vi "ResetFlowAvgFGV.vi"(9 "ignore previous (T)":bool, 10 "timeout in ms (-1)":i32=-1, 11 "Action":enum16{"Create", "Set", "Wait"}(ring)=enum."Set") -> (2 "timed out?":bool=TRUE)   [LabVIEW 2016]
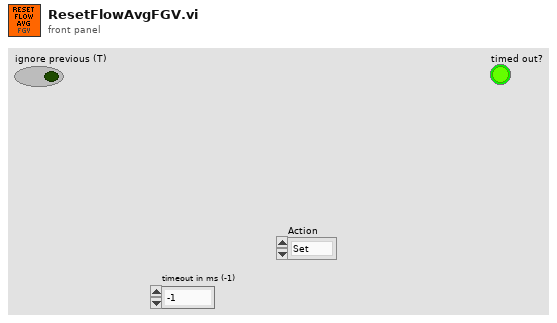
[diagram p1: front panel]
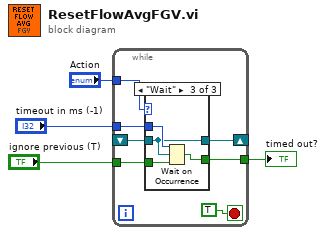
[diagram p0: block diagram]
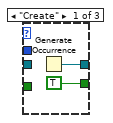
[diagram p2: hidden frame]
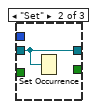
[diagram p3: hidden frame]
diagram:
  n1 = while {
    tunnel: "Action" -> [w11]
    shift-right: [w10] -> _
    shift-left: _ -> [w9]
    tunnel: "timeout in ms (-1)" -> [w8]
    tunnel: [w6] -> w2
    tunnel: "ignore previous (T)" -> [w5]
    stop <- TRUE stop-if-true
    n2 = case shown="\"Wait\"" w11 {
      tunnel: [w12 w14 w16] -> w10
      tunnel: w9 -> [_ w14 w16]
      tunnel: w8 -> [_ _ w18]
      tunnel: [TRUE ("timed out?") _ w15] -> w6
      tunnel: w5 -> [_ _ w17]
      frame "Create" {
        n3 = Generate Occurrence() -> (w12:refnum<k4>)
      }
      frame "Set" {
        n4 = Set Occurrence(w14) -> ()
      }
      frame "Wait" {
        n5 = Wait on Occurrence(1:w17, 2:w16, 3:w18) -> (0:w15:bool)
      }
    }
  }
  "timed out?" <- w2
